vi "Write Creation Date.vi"(8 "error in (no error)":errorcluster, 10 "Creation Date":timestamp, 11 "Bucket in":refnum<class "Bucket.lvclass">) -> (0 "error out":errorcluster, 3 "Bucket out":refnum<class "Bucket.lvclass">)   [LabVIEW 2015, in "NI_AWS_S3.lvlib" / "Bucket.lvclass"]
uses:
  Bucket.lvclass
  Bucket.lvclass/Bucket.ctl
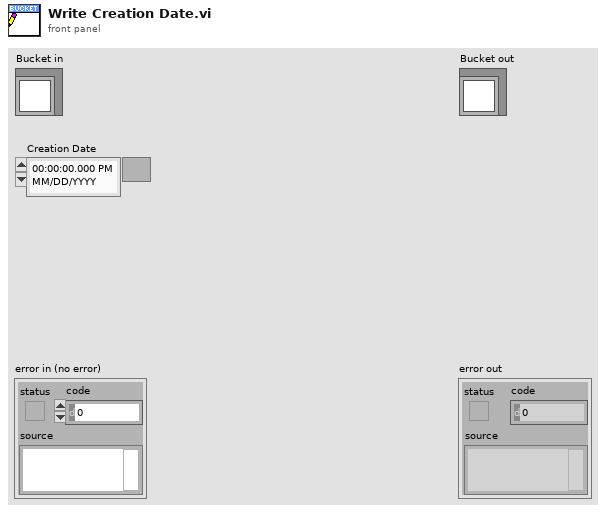
[diagram p1: front panel]
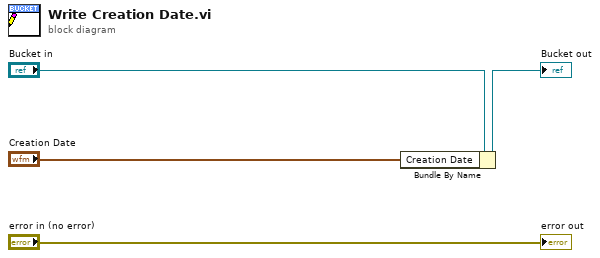
[diagram p0: block diagram]
diagram:
  n1 = Bundle By Name(cluster="Bucket in", "Creation Date"="Creation Date") -> (→"Bucket out":refnum<class "Bucket.lvclass">)
  "error out" <- "error in (no error)"
